vi "Diode-Test3-ReadAll.vi"() -> ()   [LabVIEW 2020]
panel:
  out "Live Queries":T1
  out "List of queries":T2(array[cluster])
  in  "IP Address of Device":string="192.168.203.151"
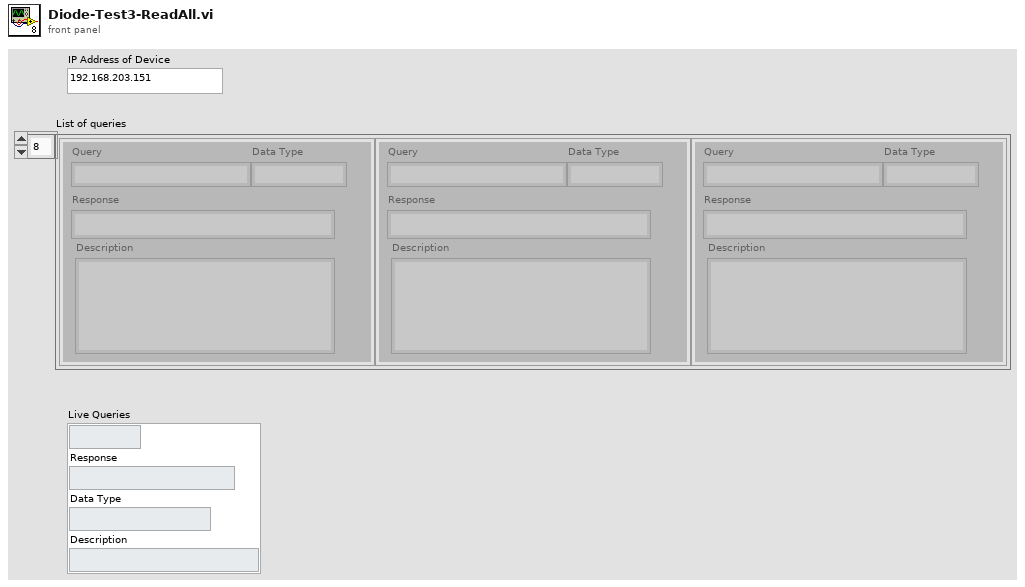
[diagram p1: front panel]
types:
  T1 = cluster{"String":string, "Response":string, "Data Type":string, "Description":string}
  T2 = cluster{"Query":string, "Response":string, "Data Type":string, "Description":string}[]
  T3 = typedef "Diode-Keyword.ctl" = cluster{"Keyword":string, "Gettable":bool, "Settable":bool, "Is Array":bool, "Data Type":string, "Description":string}
  T4 = cluster{string, "Response":string, "Is Array":bool, "Data Type":string}
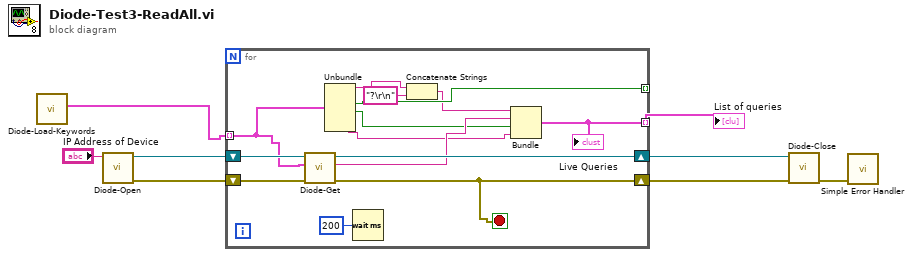
[diagram p0: block diagram]
diagram:
  n1 = call "Diode-Load-Keywords.vi"() -> ("Diodes Keywords Array"=w5:T3[])  [unwired: 11 in]
  n2 = call "Diode-Open.vi"("IP Address of Diode"="IP Address of Device") -> ("error out"=w6:errorcluster, "connection ID"=w7:refnum<k5>)  [unwired: 9 in]
  n3 = for {
    tunnel: w5 -> [w20] mode=indexing
    tunnel: [w19] -> _ mode=indexing
    shift-right: [w18] -> w4
    shift-left: w7 -> [w22]
    shift-right: [w17] -> w3
    shift-left: w6 -> [w21]
    tunnel: [w9] -> w1 mode=indexing
    stop <- w17 stop-if-true
    n4 = call "Diode-Get.vi"("error in (no error)"=w21, "Diode Keyword (leave off question mark)"=w20, "connection ID"=w22) -> ("error out"=w17:errorcluster, "Response"=w12:string, "connection ID out"=w18:refnum<k5>)  [unwired: 5 in, 1 out]
    n5 = Unbundle(w20) -> ("Keyword"=w15:string, "Settable"=w19:bool, "Is Array"=w11:bool, "Data Type"=w10:string)  [unwired: 2 out]
    n6 = Wait (ms)(milliseconds to wait=u32 200) -> ()  [unwired: 1 out]
    n7 = Concatenate Strings(w15, "?\r\n" ("string")) -> (w14:string)
    n8 = Bundle(w14, "Response"=w12, "Is Array"=w11, "Data Type"=w10) -> (w9:T4)  [unwired: 1 in]
    "Live Queries" <- w9
  }
  "List of queries" <- w1
  n9 = call "Diode-Close.vi"("error in (no error)"=w3, "connection ID"=w4) -> ("error out"=w2:errorcluster)  [unwired: 9 in]
  n10 = call <vilib>:"Simple Error Handler.vi"("error in (no error)"=w2) -> ()  [unwired: 4 in, 5 out]
